vi "Shutdown FTP Server.vi"(8 "error in (no error)":errorcluster) -> (0 "error out":errorcluster)   [LabVIEW 2017]
uses:
  ftpserve.out
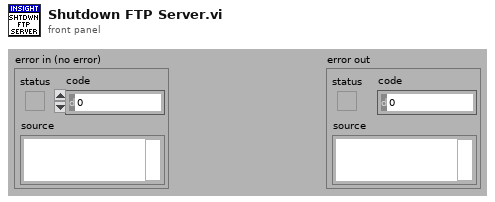
[diagram p1: front panel]
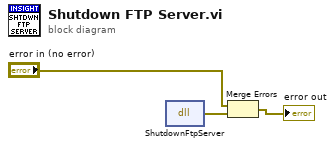
[diagram p0: block diagram]
diagram:
  n1 = dll-call lib="ftpserve.out" fn="ShutdownFtpServer"() -> (error out=w3:errorcluster)  [unwired: 4 in, 1 out]
  n2 = Merge Errors("error in (no error)", w3) -> (→"error out":errorcluster)
